vi "set owning task.vi"(10 "task":refnum<class "task.lvclass">, 11 "result in":refnum<class "result.lvclass">) -> (3 "result out":refnum<class "result.lvclass">)   [LabVIEW 2013, in "result.lvclass"]
uses:
  result.lvclass
  task/task.lvclass
  task/task.lvclass/task.ctl
  result.lvclass/result.ctl
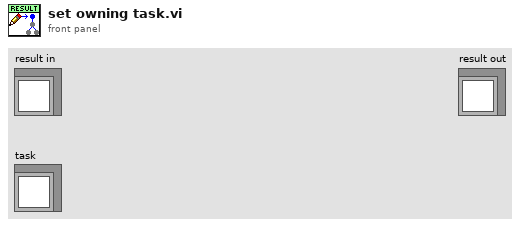
[diagram p1: front panel]
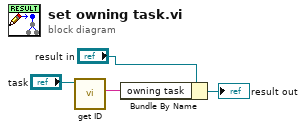
[diagram p0: block diagram]
diagram:
  n1 = call "get ID.vi"("task in"="task") -> ("ID"=w1:string)  [unwired: 9 in, 1 out]
  n2 = Bundle By Name(cluster="result in", "owning task"=w1) -> (→"result out":refnum<class "result.lvclass">)
